vi "library_variable.vi"() -> ()   [LabVIEW 2020, in "main.lvlib" / "app_data.lvlib"]
uses:
  app_data.lvlib
  app_data.ctl
panel:
  in  "app_data":refnum<data-value>
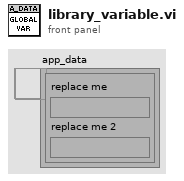
[diagram p1: front panel]
diagram:
